vi "End Autonomous.vi"   [LabVIEW 2018]
uses:
  Robot Global Data.vi
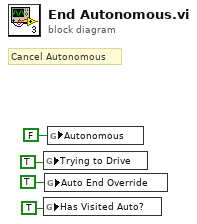
[diagram p0: block diagram]
diagram:
  # "Cancel Autonomous"
  n1 = global write "Robot Global Data.vi" "Trying to Drive"(TRUE ("Autonomous")) -> ()
  n2 = global write "Robot Global Data.vi" "Has Visited Auto?"(TRUE ("Autonomous")) -> ()
  n3 = global write "Robot Global Data.vi" "Auto End Override"(TRUE ("Autonomous")) -> ()
  n4 = global write "Robot Global Data.vi" "Autonomous"(FALSE ("Autonomous")) -> ()
